vi "HTTPMethod_Queue.vi"(4 "HttpRequestMessage":refnum<class "HttpRequestMessage.lvclass">, 5 "Queue In [create if empty]":refnum<queue>, 6 "Timeout_ms (10000)":i32=10000, 7 "Method":T1, 8 "error in (no error)":errorcluster, 9 "HttpContent":refnum<class "HttpContent.lvclass">, 10 "URL":string, 11 "LabVIEWHTTPClient_NET in":refnum<class "HttpClient_NET.lvclass">) -> (0 "error out":errorcluster, 2 "Queue Out":refnum<queue>, 3 "LabVIEWHTTPClient_NET out":refnum<class "HttpClient_NET.lvclass">)   [LabVIEW 2024, in "HttpClient_NET.lvlib" / "HttpClient_NET.lvclass"]
doc: "<b> </b> <b> </b>\nHttpClient_NET\nJustin Young - Viviota\nCopyright (c) 2021\nLicense: BSD"
uses:
  HttpClient_NET.lvclass
  HttpClient_NET.lvclass/HttpClient_NET.ctl
  Types/method_enum.ctl
  HttpClient_NET.lvlib
  HttpResponseMessage/HttpResponseMessage.lvclass
  HttpRequestMessage/HttpRequestMessage.lvclass
  HttpContent/HttpContent.lvclass
  HttpResponseMessage/Types/ResponseMessage_Cluster.ctl
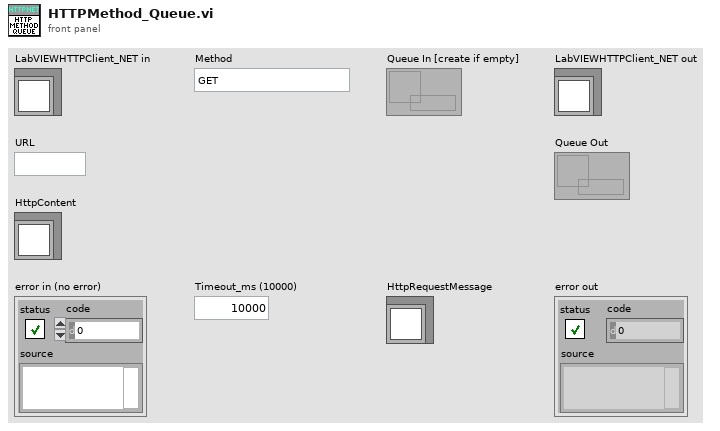
[diagram p1: front panel]
types:
  T1 = typedef "HttpClient_NET.lvlib/method_enum.ctl" = enum16{"GET", "PUT", "POST", "DELETE", "HEAD", "TRACE", "SEND"}
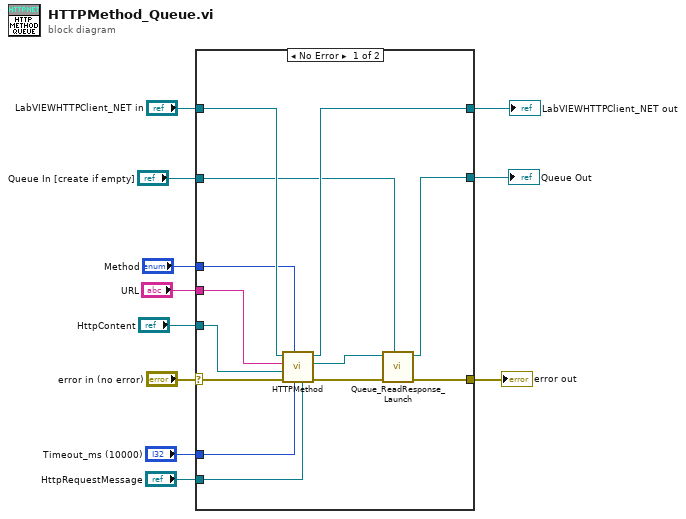
[diagram p0: block diagram]
diagram:
  n1 = case shown="No Error" "error in (no error)" {
    selector: "error in (no error)" -> [w24 w27]
    tunnel: [w13 w27] -> w10
    tunnel: [w17 w26] -> w8
    tunnel: "LabVIEWHTTPClient_NET in" -> [w21 w26]
    tunnel: "Method" -> [w20 _]
    tunnel: "Timeout_ms (10000)" -> [w23 _]
    tunnel: "URL" -> [w18 _]
    tunnel: "HttpContent" -> [w19 _]
    tunnel: "HttpRequestMessage" -> [w22 _]
    tunnel: "Queue In [create if empty]" -> [w14 w25]
    tunnel: [w12 w25] -> w1
    frame No Error {
      n2 = call "HTTPMethod.vi"("HttpRequestMessage"=w22, "Timeout_ms (10000)"=w23, "Method"=w20, "error in (no error)"=w24, "HttpContent"=w19, "URL"=w18, "LabVIEWHTTPClient_NET in"=w21) -> ("error out"=w16:errorcluster, "HttpResponseMessage out"=w15:refnum<class "HttpResponseMessage.lvclass">, "LabVIEWHTTPClient_NET out"=w17:refnum<class "HttpClient_NET.lvclass">)  [unwired: 2 in]
      n3 = call "Queue_ReadResponse_Launch.vi"("Queue In [create if empty]"=w14, "error in (no error)"=w16, "HttpResponseMessage in"=w15) -> ("error out"=w13:errorcluster, "Queue Out"=w12:refnum<queue>)  [unwired: 7 in]
    }
    frame Error {
    }
  }
  "error out" <- w10
  "LabVIEWHTTPClient_NET out" <- w8
  "Queue Out" <- w1
